vi "panel.vi"() -> ()   [LabVIEW 2023]
uses:
  <vilib>/MakerHub/LINX/Public/Peripherals/Digital/Digital Read N Chans.vi
  <vilib>/MakerHub/LINX/Public/Peripherals/Digital/Digital Write N Chans.vi
  <vilib>/MakerHub/LINX/Private/Local IO/LinxDigitalRead.vi
  <vilib>/MakerHub/LINX/Public/Utilities/Check Channel.vi
  <vilib>/MakerHub/LINX/Private/Local IO/LinxDigitalWrite.vi
  <vilib>/MakerHub/LINX/Public/Utilities/Open Serial.vi
  <vilib>/MakerHub/LINX/Private/Utilties/Generate Error.vi
  <vilib>/MakerHub/LINX/LMH-LINX.lvlib
panel:
  out "FIG_3":bool
  out "FIG_2":bool
  out "FIG_4":bool
  out "FIG_1":bool
  out "Values":bool[](array[boolean])
  in  "Serial Port":refnum<visa-resource-name>="N/A"
  in  "G7":bool
  in  "F7":bool
  in  "H7":bool
  in  "E7":bool
  in  "D7":bool
  in  "C7":bool
  in  "B7":bool
  in  "A7":bool
  in  "G6":bool
  in  "F6":bool
  in  "H6":bool
  in  "E6":bool
  in  "D6":bool
  in  "C6":bool
  in  "B6":bool
  in  "A6":bool
  in  "G5":bool
  in  "F5":bool
  in  "H5":bool
  in  "E5":bool
  in  "D5":bool
  in  "C5":bool
  in  "B5":bool
  in  "A5":bool
  in  "G4":bool
  in  "F4":bool
  in  "H4":bool
  in  "E4":bool
  in  "D4":bool
  in  "C4":bool
  in  "B4":bool
  in  "A4":bool
  in  "G3":bool
  in  "F3":bool
  in  "H3":bool
  in  "E3":bool
  in  "D3":bool
  in  "C3":bool
  in  "B3":bool
  in  "A3":bool
  in  "G2":bool
  in  "F2":bool
  in  "H2":bool
  in  "E2":bool
  in  "D2":bool
  in  "C2":bool
  in  "B2":bool
  in  "A2":bool
  in  "G1":bool
  in  "F1":bool
  in  "H1":bool
  in  "E1":bool
  in  "D1":bool
  in  "C1":bool
  in  "B1":bool
  in  "A1":bool
  in  "G0":bool
  in  "F0":bool
  in  "H0":bool
  in  "E0":bool
  in  "D0":bool
  in  "C0":bool
  in  "B0":bool
  in  "stop":bool
  in  "A0":bool
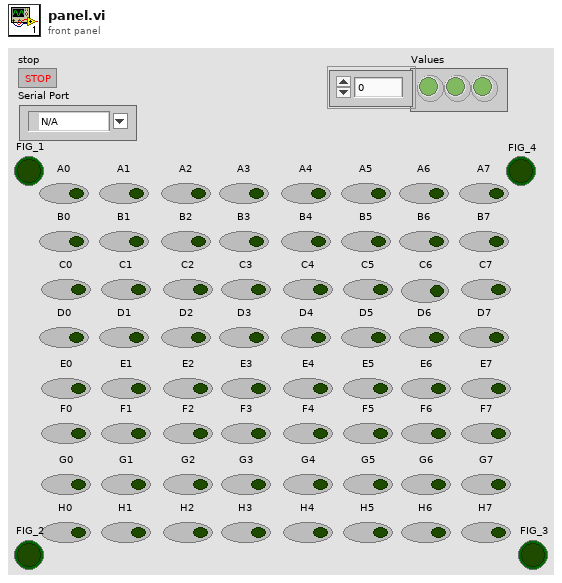
[diagram p1: front panel]
types:
  T1 = typedef "LMH-LINX.lvlib/LINX Ref.ctl" = cluster{"IO":T2, "Interface":T3, "LINX Device Config":T4}
  T2 = typedef "LMH-LINX.lvlib/Platform.ctl" = enum16{"Remote", "Local"}
  T3 = typedef "LMH-LINX.lvlib/Interface.ctl" = enum16{"Serial", "TCP"}
  T4 = typedef "LMH-LINX.lvlib/Device.lvlib/LINX Device Config.ctl" = cluster{"Interface":T3, "COM Port":refnum<visa-resource-name>, "TCP Configuration":T5, "Device Family":u8, "Device ID":u8, "Device Name":string, "TCP Ref":refnum<k5>, "Channels":T6}
  T5 = typedef "LMH-LINX.lvlib/Device.lvlib/TCP Config.ctl" = cluster{"IP Address":string, "Port":u16}
  T6 = typedef "LMH-LINX.lvlib/Channels.ctl" = cluster{"DI":u8[], "DO":u8[], "AI":u8[], "AO":u8[], "PWM":u8[], "QE":u8[], "UART":u8[], "I2C 2":u8[], "SPI":u8[], "CAN":u8[], "Servo":u8[], "AI Ref (V)":dbl, "AI Resolution (Bits)":u8, "AO Ref (V)":dbl, "AO Resolution (Bits)":u8}
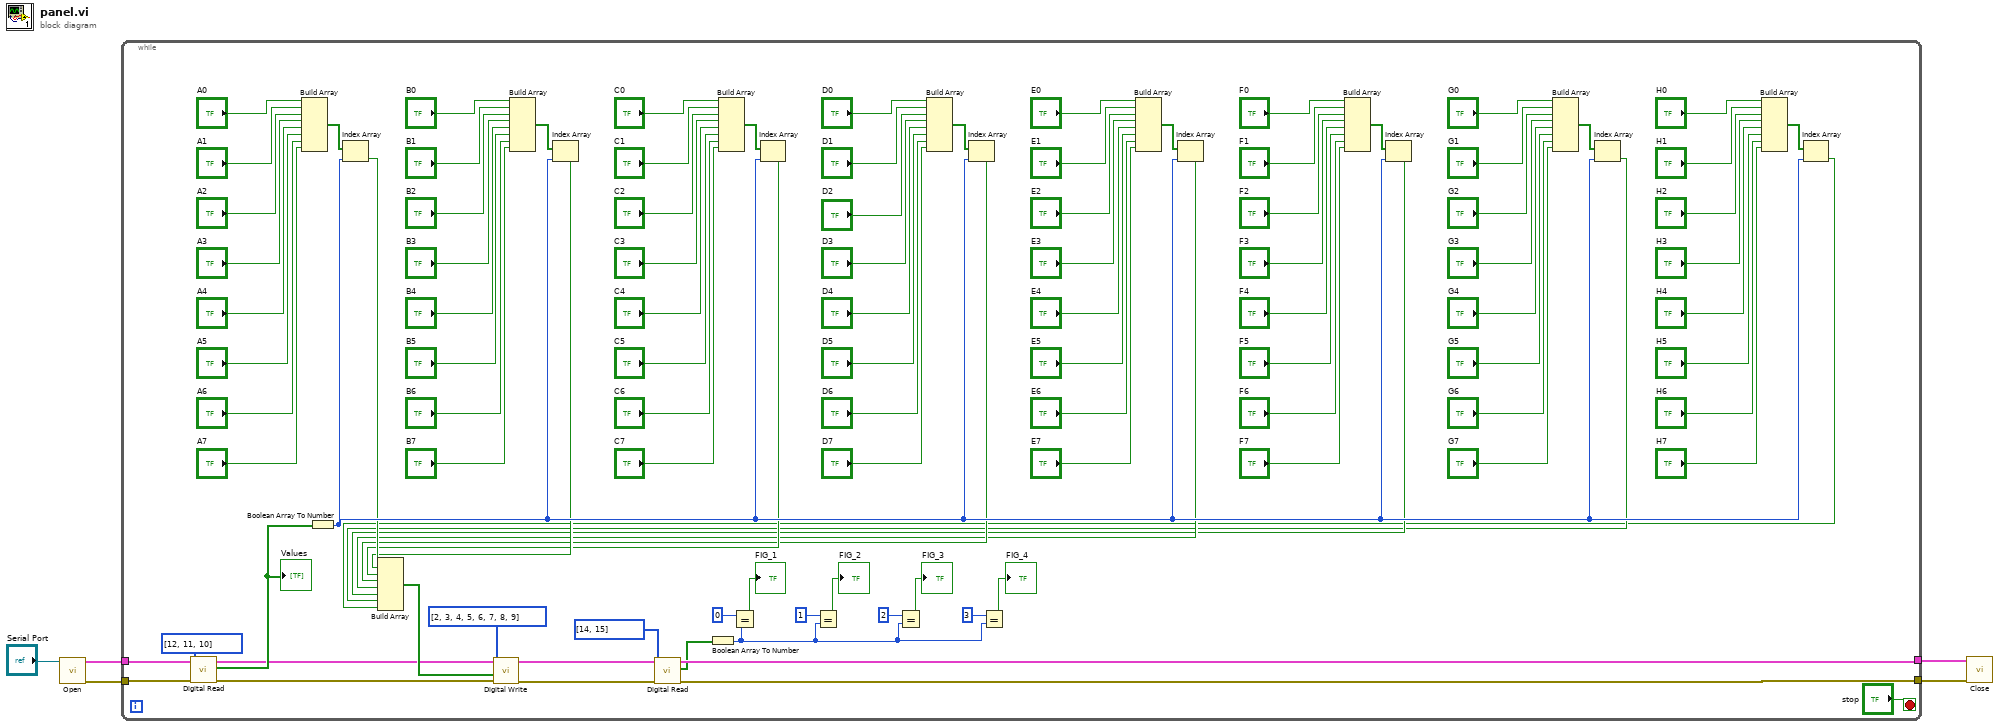
[diagram p0: block diagram]
diagram:
  n1 = call-poly <vilib>:"Open.vi"("Serial Port"="Serial Port") -> ("Error Out"=w3:errorcluster, "LINX Resource"=w4:T1)  [unwired: 8 in, 1 out]
  n2 = while {
    tunnel: w4 -> [w28]
    tunnel: w3 -> [w27]
    tunnel: [w19] -> w2
    tunnel: [w20] -> w1
    stop <- "stop" stop-if-true
    n3 = call-poly <vilib>:"Digital Read.vi"("Error In"=w27, "DI Channels"=u8[] [12, 11, 10], "LINX Resource"=w28) -> ("Error Out"=w23:errorcluster, "Values"=w26:bool[], "LINX Resource"=w24:T1)  [unwired: 6 in]
    "Values" <- w26
    n4 = Build Array("A0", "A1", "A2", "A3", "A4", "A5", "A6", "A7") -> (w45:bool[])
    n5 = Boolean Array To Number(Boolean array=w26) -> (number=w37:u32)
    n6 = Index Array(array=w45, index=w37) -> (element=w36:bool)
    n7 = Build Array("B0", "B1", "B2", "B3", "B4", "B5", "B6", "B7") -> (w44:bool[])
    n8 = Index Array(array=w44, index=w37) -> (element=w35:bool)
    n9 = Build Array("C0", "C1", "C2", "C3", "C4", "C5", "C6", "C7") -> (w43:bool[])
    n10 = Index Array(array=w43, index=w37) -> (element=w34:bool)
    n11 = Build Array("D0", "D1", "D2", "D3", "D4", "D5", "D6", "D7") -> (w42:bool[])
    n12 = Index Array(array=w42, index=w37) -> (element=w33:bool)
    n13 = Build Array("E0", "E1", "E2", "E3", "E4", "E5", "E6", "E7") -> (w41:bool[])
    n14 = Index Array(array=w41, index=w37) -> (element=w32:bool)
    n15 = Build Array("F0", "F1", "F2", "F3", "F4", "F5", "F6", "F7") -> (w40:bool[])
    n16 = Index Array(array=w40, index=w37) -> (element=w31:bool)
    n17 = Build Array("G0", "G1", "G2", "G3", "G4", "G5", "G6", "G7") -> (w39:bool[])
    n18 = Index Array(array=w39, index=w37) -> (element=w30:bool)
    n19 = Build Array("H0", "H1", "H2", "H3", "H4", "H5", "H6", "H7") -> (w38:bool[])
    n20 = Index Array(array=w38, index=w37) -> (element=w29:bool)
    n21 = Build Array(w36, w35, w34, w33, w32, w31, w30, w29) -> (w25:bool[])
    n22 = call-poly <vilib>:"Digital Write.vi"("Error In"=w23, "Values"=w25, "DO Channels"=u8[] [2, 3, 4, 5, 6, 7, 8, 9], "LINX Resource"=w24) -> ("Error Out"=w21:errorcluster, "LINX Resource"=w22:T1)  [unwired: 6 in]
    n23 = call-poly <vilib>:"Digital Read.vi"("Error In"=w21, "DI Channels"=u8[] [14, 15], "LINX Resource"=w22) -> ("Error Out"=w20:errorcluster, "Values"=w18:bool[], "LINX Resource"=w19:T1)  [unwired: 6 in]
    n24 = Boolean Array To Number(Boolean array=w18) -> (number=w10:u32)
    n25 = Equal?(x=u32 0, y=w10) -> (x = y?=→"FIG_1":bool)
    n26 = Equal?(x=u32 1, y=w10) -> (x = y?=→"FIG_2":bool)
    n27 = Equal?(x=u32 2, y=w10) -> (x = y?=→"FIG_3":bool)
    n28 = Equal?(x=u32 3, y=w10) -> (x = y?=→"FIG_4":bool)
  }
  n29 = call <vilib>:"Close.vi"("Error In"=w1, "LINX Resource"=w2) -> ()  [unwired: 9 in, 1 out]
